vi "summary results.vi"(1 "Det in use":string, 2 "Peaks":T1(array[cluster]) {"Area" format="%.4f"; "Summit Y" format="%.4f"; "End Y" format="%.4f"; "End X" format="%.4f"; "Summit X" format="%.4f"; "Start Y" format="%.4f"; "Start X" format="%.4f"}) -> (6 "summary":string[][](table), 7 "?":string[](array[string]), 8 "summary string":string)   [LabVIEW 2012]
panel:
  out "Peak times":dbl[](array[numeric]) format="%.2e"
  out "Peak areas":dbl[](array[numeric]) format="%.2e"
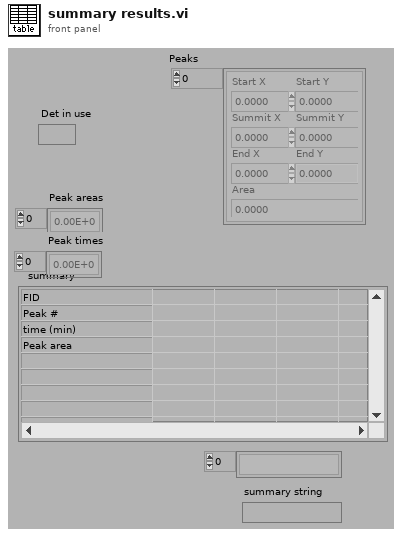
[diagram p1: front panel]
types:
  T1 = cluster{"Start X":dbl, "Start Y":dbl, "Summit X":dbl, "Summit Y":dbl, "End X":dbl, "End Y":dbl, "Area":dbl}[]
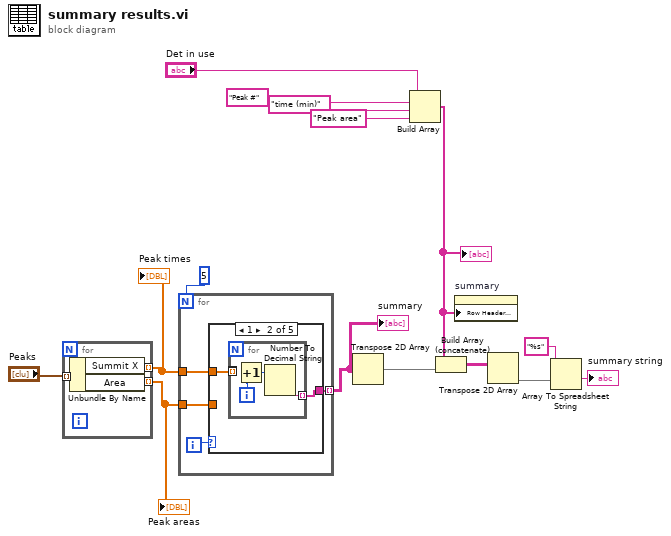
[diagram p0: block diagram]
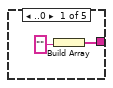
[diagram p2: hidden frame]
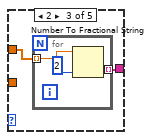
[diagram p3: hidden frame]
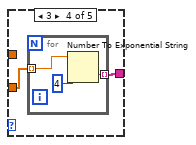
[diagram p4: hidden frame]
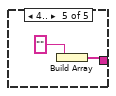
[diagram p5: hidden frame]
diagram:
  n1 = for {
    tunnel: "Peaks" -> [w18] mode=indexing
    tunnel: [w17] -> w4 mode=indexing
    tunnel: [w16] -> w3 mode=indexing
    n2 = Unbundle By Name(w18) -> ("Summit X"=w17:dbl, "Area"=w16:dbl)
  }
  "Peak areas" <- w3
  "Peak times" <- w4
  n3 = for {
    N: 5 -> [_]
    tunnel: [w21] -> w5 mode=indexing
    tunnel: w3 -> [w20]
    tunnel: w4 -> [w19]
    i -> [w22]
    n4 = case shown="1" w22 {
      tunnel: [w24 w26 w32 w37 w41] -> w21
      tunnel: w20 -> [_ _ _ w36 _]
      tunnel: w19 -> [_ w25 w31 _ _]
      frame ..0 {
        n5 = Build Array("") -> (w24:string[])
      }
      frame 1 {
        n6 = for {
          tunnel: [w29] -> w26 mode=indexing
          tunnel: [w27] -> _ mode=indexing
          tunnel: w25 -> [w27] mode=indexing
          i -> [w30]
          n7 = Increment(x=w30) -> (x+1=w28:i32)
          n8 = Number To Decimal String(number=w28) -> (decimal integer string=w29:string)  [unwired: 1 in]
        }
      }
      frame 2 {
        n9 = for {
          tunnel: w31 -> [w35] mode=indexing
          tunnel: [w33] -> w32 mode=indexing
          n10 = Number To Fractional String(number=w35, precision (6)=2) -> (F-format string=w33:string)  [unwired: 2 in]
        }
      }
      frame 3 {
        n11 = for {
          tunnel: w36 -> [w40] mode=indexing
          tunnel: [w39] -> w37 mode=indexing
          n12 = Number To Exponential String(number=w40, precision (6)=4) -> (E-format string=w39:string)  [unwired: 2 in]
        }
      }
      frame 4.. {
        n13 = Build Array("") -> (w41:string[])
      }
    }
  }
  "summary" <- w5
  n14 = Transpose 2D Array(2D array=w5) -> (transposed array=w13:string[][])
  n15 = Build Array("Det in use", "Peak #", "time (min)", "Peak area") -> (w7:string[])
  "?" <- w7
  n16 = Build Array (concatenate)(w7, w13) -> (w12:string[][])
  n17 = property on="summary" class="Tbl (strict)"("Row Header Strings[]"=w7) -> ()  [unwired: 2 in, 2 out]
  n18 = Transpose 2D Array(2D array=w12) -> (transposed array=w11:string[][])
  n19 = Array To Spreadsheet String(array=w11, 3:"%s") -> (spreadsheet string=→"summary string":string)  [unwired: 1 in]
